vi "_RT_CtrlLoop_D999_Conv_AO_Value.vi"(1 "valid":bool, 3 "Response Str":string) -> (0 "AO Array":i32[](array[numeric]))   [LabVIEW 2018]
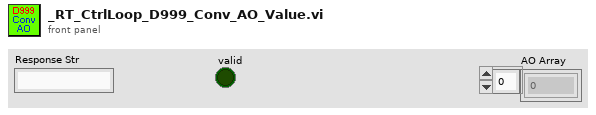
[diagram p1: front panel]
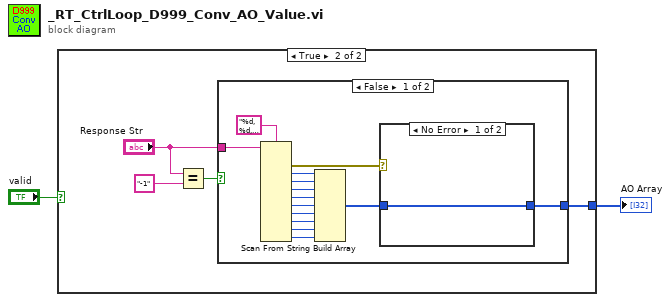
[diagram p0: block diagram]
diagram:
  n1 = case shown="True" "valid" {
    tunnel: [_ w6] -> w1
    frame False {
    }
    frame True {
      n2 = Equal?(x="Response Str", y="-1") -> (x = y?=w3:bool)
      n3 = case shown="False" w3 {
        tunnel: [w8 _] -> w6
        tunnel: "Response Str" -> [w7 _]
        frame False {
          n4 = Scan From String(format string="%d,%d,%d,%d,%d,%d,%d,%d,%d", input string=w7) -> (error out=w10:errorcluster, output 1=w13:i32, output 2=w14:i32, output 3=w15:i32, output 4=w16:i32, output 5=w17:i32, output 6=w18:i32, output 7=w19:i32, output 8=w20:i32, output 9=w11:i32)  [unwired: 11 in, 2 out]
          n5 = Build Array(w13, w14, w15, w16, w17, w18, w19, w20, w11) -> (w9:i32[])
          n6 = case shown="No Error" w10 {
            tunnel: w9 -> [w21 _]
            tunnel: [w21 _] -> w8
            frame No Error {
            }
            frame Error {
            }
          }
        }
        frame True {
        }
      }
    }
  }
  "AO Array" <- w1
